vi "Formulanode.vi"() -> ()   [LabVIEW 2020]
doc: "This VI is a solution to an exercise in the LabVIEW Basics I course.\n\nThis VI uses the Formula Node to evaluate the following equation:\n y = a**3 + a where a = tanh (x) + cos (x)"
panel:
  out "Waveform Graph":dbl[](graph)
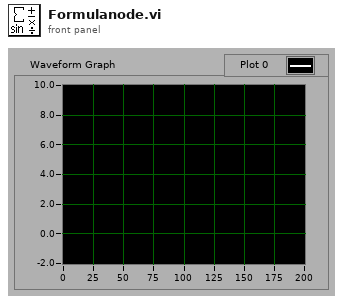
[diagram p1: front panel]
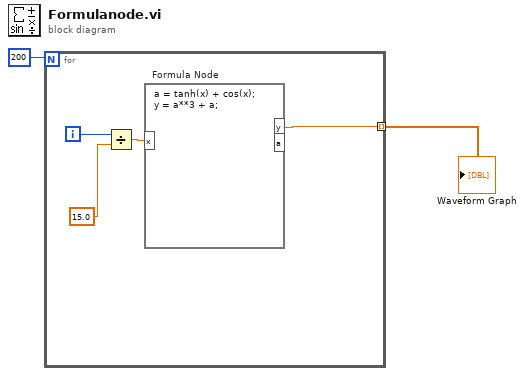
[diagram p0: block diagram]
diagram:
  n1 = for {
    N: 200 -> [_]
    tunnel: [w5] -> w1 mode=indexing
    i -> [w4]
    n2 = Divide(x=w4, y=15.0) -> (x/y=w6:dbl)
    n3 = formula code="a = tanh(x) + cos(x);\ny = a**3 + a;"("x"=w6) -> ("y"=w5:dbl)  [unwired: 1 out]
  }
  "Waveform Graph" <- w1
